vi "goal_check.vi"(4 "flag":i32, 5 "table":i32[](array[numeric])) -> (0 "fin":bool, 1 "win step":i32[](array[numeric]), 2 "empty":i32[](array[numeric]))   [LabVIEW 8.6]
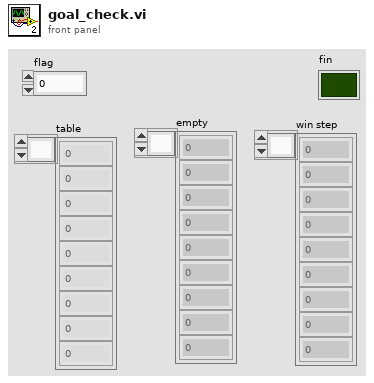
[diagram p1: front panel]
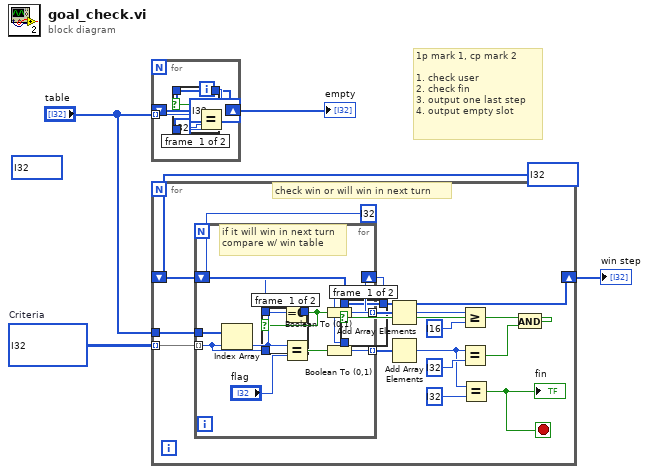
[diagram p0: block diagram]
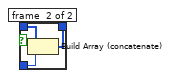
[diagram p2: hidden frame]
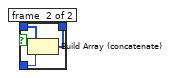
[diagram p3: hidden frame]
diagram:
  (unwired) i32[] ? ("table 2")
  w3 = i32[][] ?  # Criteria
  # "1p mark 1, cp mark 2\n\n1. check user\n2. check fin\n3. output one last step\n4. output empty slot"
  n1 = for {
    tunnel: "table" -> [w11] mode=indexing
    shift-right: [w7] -> w5
    shift-left: i32[] ? ("Array") -> [w8]
    i -> [w9]
    n2 = Equal?(x=w11, y=i32 ?) -> (x = y?=w10:bool)
    n3 = case shown="True" w10 {
      tunnel: w8 -> [w13 w15]
      tunnel: w9 -> [_ w14]
      tunnel: [w13 w16] -> w7
      frame #0 {
      }
      frame #1 {
        n4 = Build Array (concatenate)(w15, w14) -> (w16:i32[])
      }
    }
  }
  "empty" <- w5
  n5 = for {
    tunnel: w3 -> [w32] mode=indexing
    tunnel: "table" -> [w33]
    shift-right: [w18] -> w4
    shift-left: i32[] ? ("Array") -> [w19]
    stop <- w20 stop-if-true
    # "check win or will win in next turn"
    n6 = for {
      tunnel: w33 -> [w47]
      tunnel: w32 -> [w43] mode=indexing
      tunnel: [w44] -> w27 mode=indexing
      tunnel: [w41] -> w25 mode=indexing
      shift-right: [w38] -> w28
      shift-left: i32 ? ("Numeric") -> [w39]
      # "if it will win in next turn\ncompare w/ win table"
      n7 = Index Array(array=w47, index=w43) -> (element=w42:i32)
      n8 = Equal To 0?(x=w42) -> (x = 0?=w40:bool)
      n9 = case shown="True" w40 {
        tunnel: w39 -> [w48 _]
        tunnel: w43 -> [_ w49]
        tunnel: [w48 w49] -> w38
        frame #0 {
        }
        frame #1 {
        }
      }
      n10 = Equal?(x=w42, y="flag") -> (x = y?=w45:bool)
      n11 = Boolean To (0,1)(Boolean=w40) -> (0, 1=w41:i16)
      n12 = Boolean To (0,1)(Boolean=w45) -> (0, 1=w44:i16)
    }
    n13 = Add Array Elements(numeric array=w25) -> (sum=w24:i16)
    n14 = Add Array Elements(numeric array=w27) -> (sum=w29:i16)
    n15 = Greater Or Equal?(x=w24, y=i16 ?) -> (x >= y?=w22:bool)
    n16 = Equal?(x=w29, y=i32 ? ("index")) -> (x = y?=w26:bool)
    n17 = Equal?(x=w29, y=i32 ? ("index")) -> (x = y?=w20:bool)
    "fin" <- w20
    n18 = And(x=w22, y=w26) -> (x .and. y?=w21:bool)
    n19 = case shown="True" w21 {
      tunnel: w19 -> [w34 w36]
      tunnel: w28 -> [_ w35]
      tunnel: [w34 w37] -> w18
      frame #0 {
      }
      frame #1 {
        n20 = Build Array (concatenate)(w36, w35) -> (w37:i32[])
      }
    }
  }
  "win step" <- w4
